vi "dvp Vi Set Timer Value.vi"(10 "TimerValue":dbl, 11 "handle":u32) -> (3 "function return":u32(ring))   [LabVIEW 2018, in "LabViewDVPCamera.lvlib"]
doc: "LabviewDvp2Api dvpStatus dvpViSetTimerValue(dvpHandle handle, double TimerValue);"
uses:
  LabViewDVPCamera.lvlib
  LabViewDVPCamera/LabViewDVPCamera.dll
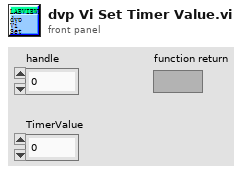
[diagram p1: front panel]
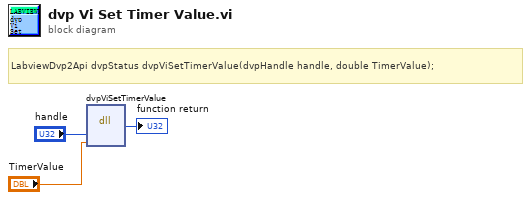
[diagram p0: block diagram]
diagram:
  # "LabviewDvp2Api dvpStatus dvpViSetTimerValue(dvpHandle handle, double TimerValue);"
  n1 = dll-call lib="C:/Program Files (x86)/DVP2 Labview cn 64/Sample/LabViewDVPCamera/LabViewDVPCamera.*" fn="dvpViSetTimerValue"("handle"="handle", "TimerValue"="TimerValue") -> (→"function return":u32)  [unwired: 5 in, 2 out]
